vi "PVCamGlobalVariables.vi"() -> ()   [LabVIEW 2019]
panel:
  out "Histogram Enabled":bool
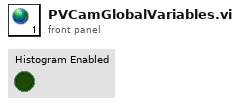
[diagram p1: front panel]
diagram:
